vi "GetMessage.vi"(0 "reference in":refnum<class "Device.lvclass">, 2 "Sender":string, 5 "error in (no error)":errorcluster, 8 "Message":string) -> (14 "reference out":refnum<class "Device.lvclass">, 19 "error out":errorcluster)   [LabVIEW 2013, in "Device.lvclass"]
uses:
  Device.lvclass
  Colleague_class/Colleague.lvclass
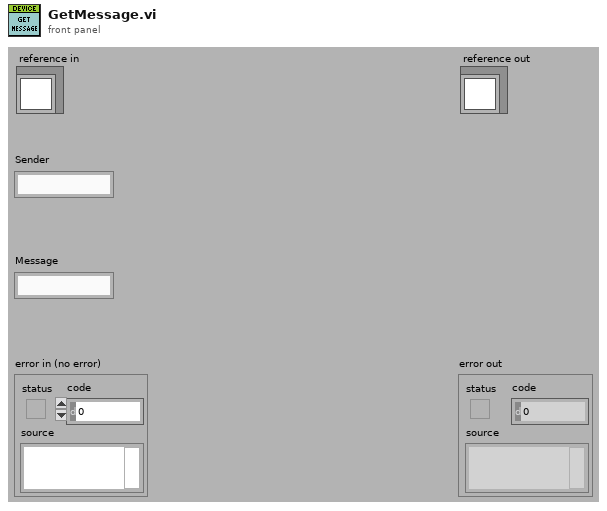
[diagram p1: front panel]
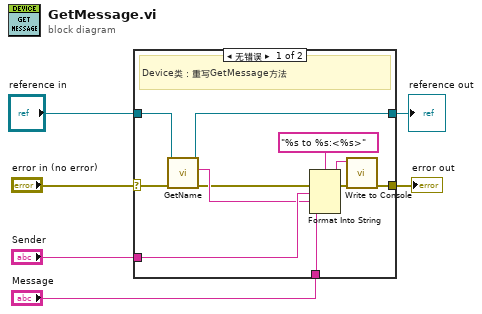
[diagram p0: block diagram]
diagram:
  n1 = case shown="无错误" "error in (no error)" {
    selector: "error in (no error)" -> [w11 w19]
    tunnel: [w7 w19] -> w5
    tunnel: [w16 w18] -> w3
    tunnel: "reference in" -> [w17 w18]
    tunnel: "Sender" -> [w14 _]
    tunnel: "Message" -> [w12 _]
    frame No Error {
      # "Device类：重写GetMessage方法"
      n2 = call "GetName.vi"("error in (no error)"=w11, "reference in"=w17) -> ("error out"=w10:errorcluster, "Name"=w13:string, "reference out"=w16:refnum<class "Device.lvclass">)  [unwired: 7 in]
      n3 = Format Into String(format string="%s to %s:<%s>" ("格式字符串"), error in=w10, w14, w13, w12) -> (resulting string=w8:string, error out=w9:errorcluster)  [unwired: 1 in]
      n4 = call "Write to Console.vi"("error in (no error)"=w9, "Input"=w8) -> ("error out"=w7:errorcluster)  [unwired: 9 in]
    }
    frame Error {
    }
  }
  "error out" <- w5
  "reference out" <- w3
